vi "Export time-lapse images-path management.vi"(11 "AVI path in":path) -> (1 "cancelled":bool, 2 "New folder path":path, 3 "Existing AVI path":path)   [LabVIEW 2013]
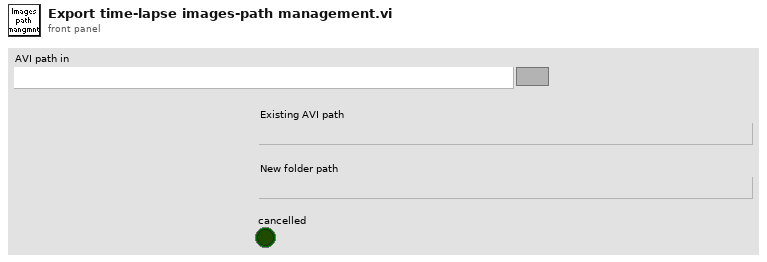
[diagram p1: front panel]
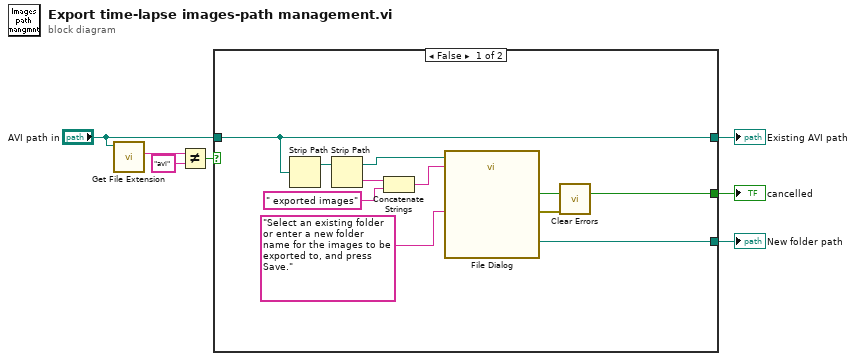
[diagram p0: block diagram]
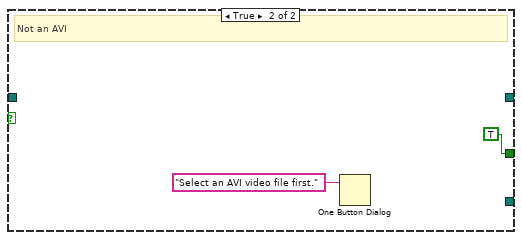
[diagram p2: hidden frame]
diagram:
  n1 = call <vilib>:"Get File Extension.vi"("file"="AVI path in") -> ("lowercase file extension"=w2:string)  [unwired: 7 in, 3 out]
  n2 = Not Equal?(x=w2, y="avi") -> (x != y?=w4:bool)
  n3 = case shown="False" w4 {
    tunnel: [w15 _] -> w6
    tunnel: [w17 TRUE ("cancelled")] -> w5
    tunnel: "AVI path in" -> [w15 _]
    tunnel: [w16 _] -> w7
    frame False {
      n4 = Strip Path(path=w15) -> (stripped path=w14:path)  [unwired: 1 out]
      n5 = Strip Path(path=w14) -> (stripped path=w11:path, name=w13:string)
      n6 = Concatenate Strings(w13, " exported images" ("format string")) -> (w9:string)
      n7 = call "File Dialog"("start path"=w11, "prompt"="Select an existing folder or enter a new folder name for the images to be exported to, and press Save.", "default name"=w9) -> ("selected path"=w16:path, "cancelled"=w17:bool, "error out"=w10:errorcluster)  [unwired: 9 in, 1 out]
      n8 = call <vilib>:"Clear Errors.vi"("error in (no error)"=w10) -> ()  [unwired: 6 in, 1 out]
    }
    frame True {
      # "Not an AVI"
      n9 = One Button Dialog(message="Select an AVI video file first.") -> ()  [unwired: 1 in, 1 out]
    }
  }
  "New folder path" <- w7
  "Existing AVI path" <- w6
  "cancelled" <- w5
